vi "Not Openable VI Message.vi"() -> ()   [LabVIEW 2020, in "Peek Window.lvlib" / "Standard VI Type.lvclass"]
uses:
  Standard VI Type.lvclass
panel:
  out "VI Full Qualified Name":string
  # "Unable to display selected VI's Block Diagram."
  # "Possible reasons:\n\nIt may already be open in another window.\nIt may be password-protected.\nIt may have been saved with its diagram removed."
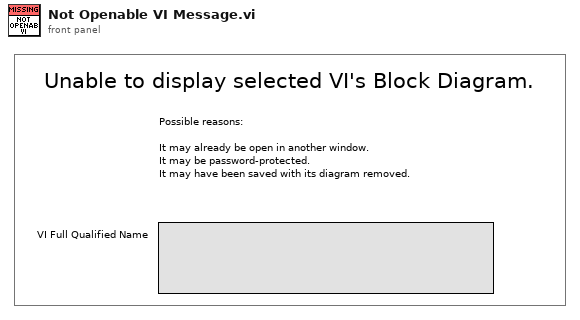
[diagram p1: front panel]
diagram:
